vi "LVFunction_Imop_SlopesPostProcessor_Apply ShutOfBoundaries.vi"(0 "HasoSlopes in":refnum<class "HasoSlopes.lvclass">, 5 "HasoSlopes OUT":refnum<class "HasoSlopes.lvclass">, 7 "ShutOfBoundaries":u32, 11 "error in (no error)":errorcluster) -> (4 "HasoSlopes out":refnum<class "HasoSlopes.lvclass">, 6 "HasoSlopes OUT 2":refnum<class "HasoSlopes.lvclass">, 15 "error out":errorcluster)   [LabVIEW 2020]
uses:
  HasoSlopes.lvclass
  LVClass_HasoSlopes Read HasoSlopes _ property.vi
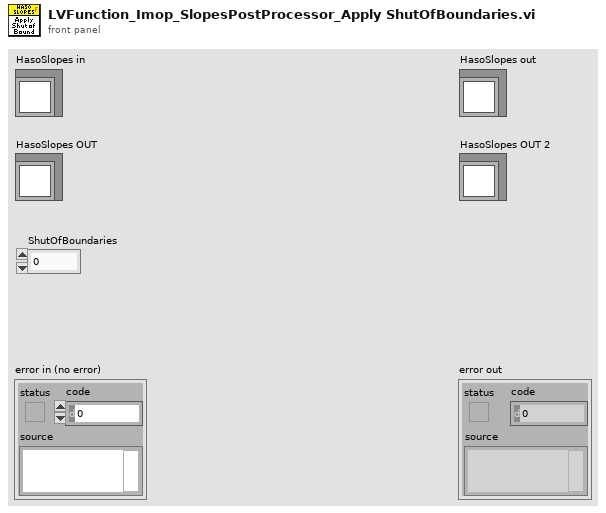
[diagram p1: front panel]
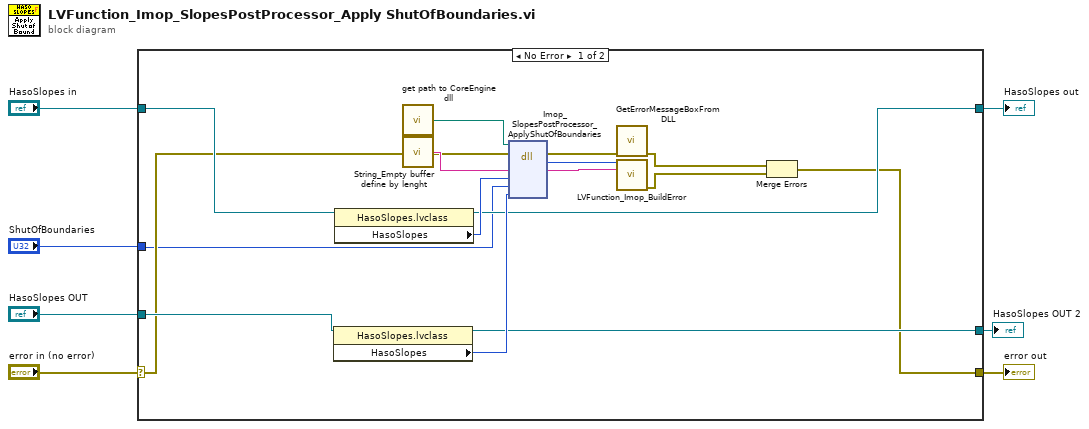
[diagram p0: block diagram]
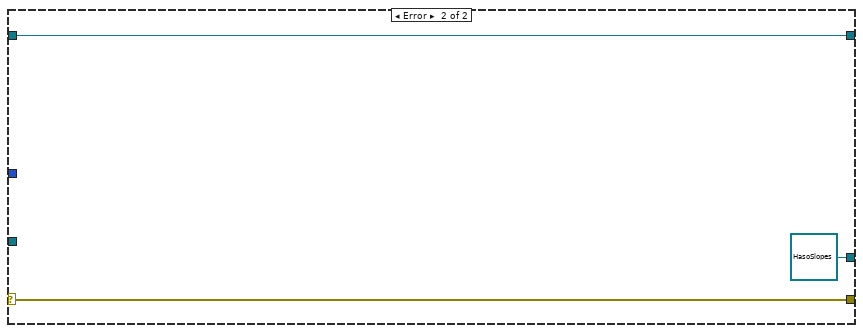
[diagram p2: hidden frame]
diagram:
  n1 = case shown="No Error" "error in (no error)" {
    selector: "error in (no error)" -> [w10 w26]
    tunnel: [w9 w26] -> w6
    tunnel: [w12 w25] -> w4
    tunnel: "HasoSlopes in" -> [w13 w25]
    tunnel: "HasoSlopes OUT" -> [w14 _]
    tunnel: [w11 refnum<class "HasoSlopes.lvclass"> refnum ("HasoSlopes OUT")] -> w2
    tunnel: "ShutOfBoundaries" -> [w8 _]
    frame No Error {
      n2 = property class="HasoSlopes.lvclass"(reference=w14) -> (reference out=w11:refnum<class "HasoSlopes.lvclass">, "HasoSlopes"=w15:i32)  [unwired: 1 in, 1 out]
      n3 = property class="HasoSlopes.lvclass"(reference=w13) -> (reference out=w12:refnum<class "HasoSlopes.lvclass">, "HasoSlopes"=w23:i32)  [unwired: 1 in, 1 out]
      n4 = call "get path to CoreEngine dll.vi"() -> ("path to c_interface_vc100.dll"=w18:path)  [unwired: 12 in, 3 out]
      n5 = call "String_Empty buffer define by lenght.vi"() -> ("Empty buffer"=w19:string)  [unwired: 1 in]
      n6 = dll-call lib="D:/FLE/0.Code/CoreEngine4_Suite/LV2011_interface/DLLs/c_interface_vc100.dll" fn="Imop_SlopesPostProcessor_ApplyShutOfBoundaries"(path in=w18, error in=w10, "Message"=w19, "HasoSlopes IN"=w23, "Shut of boundaries"=w8, "HasoSlopes OUT"=w15) -> (error out=w22:errorcluster, "return type"=w20:i32, "Message"=w21:string)  [unwired: 4 in, 1 out]
      n7 = call "GetErrorMessageBoxFromDLL.vi"("error IN"=w22) -> ("error OUT"=w17:errorcluster)  [unwired: 10 in]
      n8 = call "LVFunction_Imop_BuildError.vi"("code"=w20, "String to Prepend to source (\"\")"=w21) -> ("error out"=w16:errorcluster)  [unwired: 13 in]
      n9 = Merge Errors(w17, w16) -> (w9:errorcluster)
    }
    frame Error {
    }
  }
  "error out" <- w6
  "HasoSlopes out" <- w4
  "HasoSlopes OUT 2" <- w2
